vi "Get Slope of Array between points.vi"() -> ()   [LabVIEW 2012]
uses:
  <vilib>/Analysis/NI_AAL_SigProc.lvlib
panel:
  out "Slope of Line (points skipped =3)":cluster{dbl[], dbl[]}(graph)
  out "Locations":dbl[](array[numeric])
  out "time":dbl[](array[numeric])
  out "Waveform Graph 2":dbl[](graph)
  out "Waveform Graph":dbl[](graph)
  out "power":dbl[](array[numeric])
  out "time sub":dbl[](array[numeric])
  in  "time":dbl[](array[numeric])=[0.0, 160.80188751220703, 319.5328712463379, 479.2613983154297, 639.4448280334473, 798.926830291748, 959.9084854125977, 1118.4439659118652, 1278.6788940429688, 1438.7798309326172, 1599.4839668273926, 1757.883071899414, 1917.273998260498, 2077.633857727051, 2237.741470336914, 2397.1524238586426, 2556.86092376709, 2717.7953720092773, 2876.4801025390625, 3036.529541015625, 3196.6781616210938, 3356.1763763427734, 3516.683578491211, 3675.765037536621, 3836.2832069396973, 3994.917392730713, 4155.839443206787, 4316.474437713623, 4475.836753845215, 4634.658336639404, 4795.10498046875, 4954.459190368652, 5115.270614624023, 5274.047374725342, 5433.9470863342285, 5594.878196716309, 5753.260612487793, 5913.294315338135, 6073.932647705078, 6232.86771774292, 6392.690658569336, 6554.119110107422, 6712.586879730225, 6873.498439788818, 7032.4506759643555, 7287.8875732421875, 7448.5578536987305, 7607.880115509033, 7767.521381378174, 7927.871227264404, 8088.170528411865, 8247.288703918457, 8406.580924987793, 8566.125869750977, 8726.202964782715, 8886.642456054688, 9046.812534332275, 9205.270767211914, 9365.05937576294, 9525.272846221924, 9686.171054840088, 9845.497608184814, 10004.202842712402, 10163.961410522461, 10323.89497756958, 10484.039783477783, 10645.226955413818, 10804.120540618896, 10963.831901550293, 11123.775005340576, 11283.164978027344, 11444.32020187378, 11603.68824005127, 11762.360095977783, 11921.841144561768, 12082.343578338623, 12243.229866027832, 12401.914119720459, 12561.808109283447, 12722.314834594727, 12881.348133087158, 13041.152000427246, 13201.125144958496, 13360.804080963135, 13521.149158477783, 13681.74934387207, 13840.245723724365, 13999.918937683105, 14255.95235824585, 14415.825843811035, 14575.607776641846, 14735.746383666992, 14896.51346206665, 15054.931640625]
  out "appended array":dbl[](array[numeric])
  out "Arrayin":dbl[](array[numeric])
  in  "Number of points":i32
  in  "Array of values":dbl[](array[numeric])
  out "Array of slopes":dbl[](array[numeric])
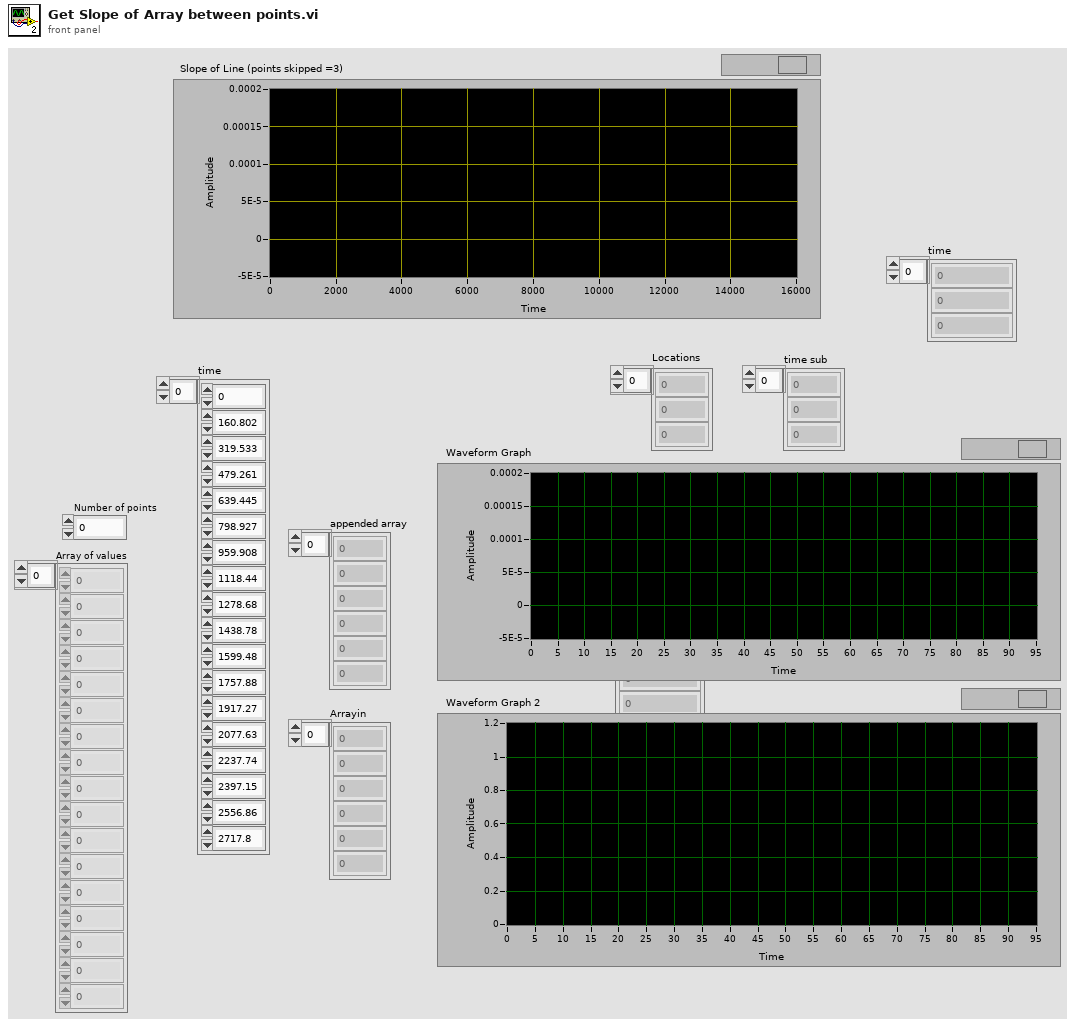
[diagram p1: front panel]
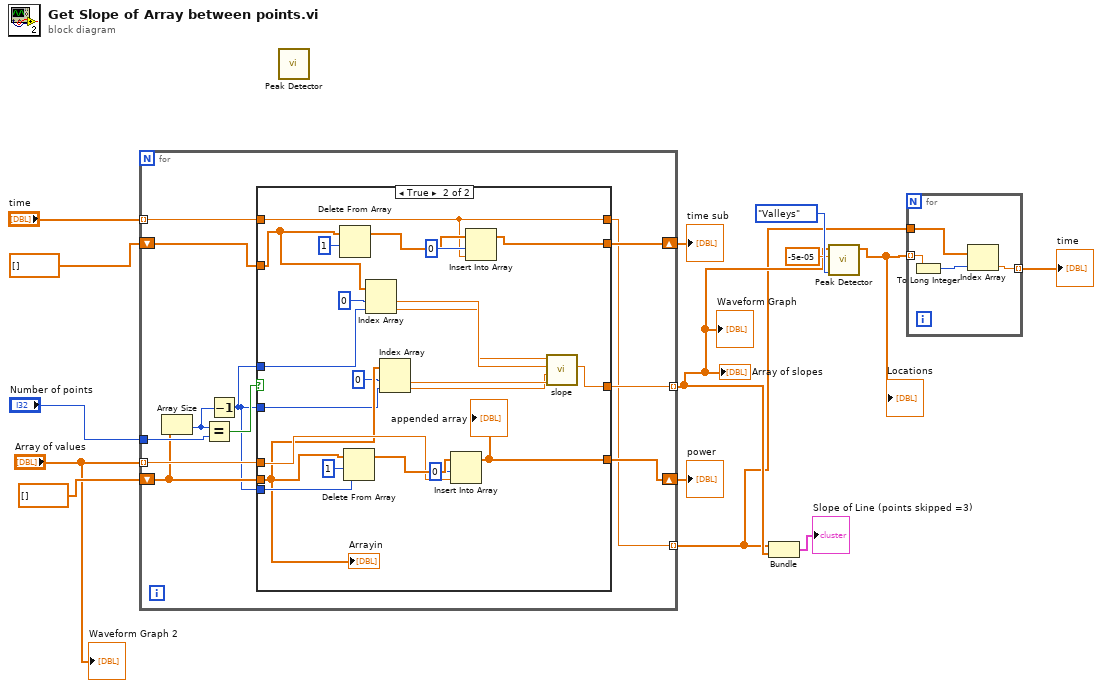
[diagram p0: block diagram]
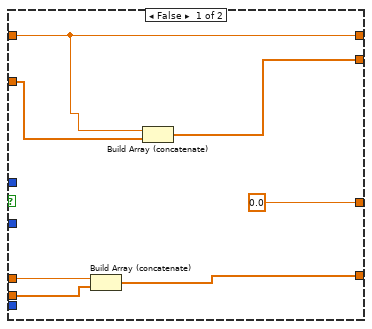
[diagram p2: hidden frame]
diagram:
  n1 = for {
    tunnel: "Array of values" -> [w24] mode=indexing
    tunnel: "Number of points" -> [w26]
    shift-right: [w23] -> w10
    shift-left: dbl[] [] ("Array of averages") -> [w21]
    tunnel: [w22] -> w3 mode=indexing
    tunnel: "time" -> [w19] mode=indexing
    shift-right: [w17] -> w5
    shift-left: dbl[] [] ("Array of averages") -> [w18]
    tunnel: [w15] -> w1 mode=indexing
    n2 = Array Size(array=w21) -> (size(s)=w20:i32)
    n3 = Equal?(x=w20, y=w26) -> (x = y?=w25:bool)
    n4 = Decrement(x=w20) -> (x-1=w16:i32)
    n5 = case shown="True" w25 {
      tunnel: w24 -> [w33 w53]
      tunnel: w21 -> [w32 w49]
      tunnel: [w31 w51] -> w23
      tunnel: [0.0 ("mean") w35] -> w22
      tunnel: w16 -> [_ w50]
      tunnel: w19 -> [w28 w34]
      tunnel: [w28 w34] -> w15
      tunnel: w18 -> [w29 w38]
      tunnel: [w27 w44] -> w17
      tunnel: w16 -> [_ w43]
      tunnel: w16 -> [_ w39]
      frame False {
        n6 = Build Array (concatenate)(w33, w32) -> (w31:dbl[])
        n7 = Build Array (concatenate)(w28, w29) -> (w27:dbl[])
      }
      frame True {
        n8 = Delete From Array(array=w38, length=1) -> (array with subset deleted=w46:dbl[])  [unwired: 1 in, 1 out]
        n9 = Delete From Array(array=w49, length=1, index=w50) -> (array with subset deleted=w54:dbl[])  [unwired: 1 out]
        n10 = Index Array(array=w38, index #1=0 ("index"), index #2=w39) -> (element #1=w37:dbl, element #2=w36:dbl)
        n11 = Index Array(array=w49, index #1=0 ("index"), index #2=w43) -> (element #1=w42:dbl, element #2=w41:dbl)
        n12 = Insert Into Array(array=w54, index=0, new element=w53) -> (w51:dbl[])
        "appended array" <- w51
        n13 = Insert Into Array(array=w46, index=0, new element=w34) -> (w44:dbl[])
        n14 = call "slope.vi"("y 2"=w42, "y1"=w41, "x 2"=w37, "x1"=w36) -> ("Slope"=w35:dbl)  [unwired: 7 in]
        "Arrayin" <- w49
      }
    }
  }
  "Array of slopes" <- w3
  "time sub" <- w5
  "power" <- w10
  "Waveform Graph" <- w3
  n15 = call <vilib>:"Peak Detector.vi"() -> ()  [unwired: 7 in, 5 out]
  n16 = Bundle(w1, w3) -> (→"Slope of Line (points skipped =3)":cluster{dbl[], dbl[]})  [unwired: 1 in]
  n17 = call <vilib>:"Peak Detector.vi"("peaks/valleys"=enum32{"Peaks", "Valleys"}."Valleys", "threshold"=-5e-05, "X"=w3) -> ("Locations"=w6:dbl[])  [unwired: 4 in, 4 out]
  "Locations" <- w6
  n18 = for {
    tunnel: w6 -> [w56] mode=indexing
    tunnel: w1 -> [w59]
    tunnel: [w58] -> w4 mode=indexing
    n19 = To Long Integer(number=w56) -> (32bit integer=w57:i32)
    n20 = Index Array(array=w59, index=w57) -> (element=w58:dbl)
  }
  "time" <- w4
  "Waveform Graph 2" <- "Array of values"
